vi "cycleAllNLMethods_invP.vi"() -> ()   [LabVIEW 2014]
uses:
  ICRMKinematics.llb/nloptIKParams.ctl
  02_optimalHome/homeBus.ctl
  ICRMKinematics.llb/jntLims.ctl
  CWrapATC3DG/Release/CWrapATC3DG.llb/ascSetup.ctl
  <vilib>/Analysis/Matrix/Datatypes/RealMatrix.ctl
  ICRMKinematics.llb/knPms11A.ctl
  <vilib>/Analysis/Matrix/NI_Matrix.lvlib
panel:
  out "results":T3(array[cluster])=[{"invParams"={"nlParams"={"maxIts"=100000.0, "maxTimeSec"=60.0, "nlMethod"=enum."GN_DIRECT", "errTol"=1e-09, "tolFun"=1e-09, "tolX"=1e-09}, "qp0"=[0.0, 0.0, 0.0, 1.0, 100.0], "q0dn"=[-0.4, -0.2, -0.2, -0.2, -10.0], "q0up"=[0.4, 0.2, 0.2, 0.2, 10.0], "kn0"={"tx01"=806.0, "ty01"=-66.0, "tz01"=-28.0, "ry01"=0.0, "rz01"=-0.24, "tx23"=8.2, "ry34"=0.0, "rz34"=0.0, "cathL"=98.0, "ry45"=0.0, "rz45"=0.0}, "knPM"={"tx01"=20.0, "ty01"=20.0, "tz01"=20.0, "ry01"=0.2, "rz01"=0.2, "tx23"=1.0, "ry34"=0.2, "rz34"=0.2, "cathL"=10.0, "ry45"=0.2, "rz45"=0.2}}, "qps0out"=[-0.014814814700095935, -0.0666666667240261, 0.06666666660930724, -0.19999999994264056, -3.3333333304653614], "kn"={"tx01"=820.7873799668292, "ty01"=-46.00000000573594, "tz01"=-8.000000005735945, "ry01"=-0.022222222164862783, "rz01"=-0.2029629629056035, "tx23"=9.199999999713203, "ry34"=0.19999999994264056, "rz34"=-0.19999999994264056, "cathL"=88.00000000286798, "ry45"=-0.007407407350047968, "rz45"=-0.06666666683874499}, "fmin"=78538.53053676435, "retCodeOut"=3}, {"invParams"={"nlParams"={"maxIts"=100000.0, "maxTimeSec"=60.0, "nlMethod"=enum."GN_DIRECT_L", "errTol"=1e-09, "tolFun"=1e-09, "tolX"=1e-09}, "qp0"=[0.0, 0.0, 0.0, 1.0, 100.0], "q0dn"=[-0.4, -0.2, -0.2, -0.2, -10.0], "q0up"=[0.4, 0.2, 0.2, 0.2, 10.0], "kn0"={"tx01"=806.0, "ty01"=-66.0, "tz01"=-28.0, "ry01"=0.0, "rz01"=-0.24, "tx23"=8.2, "ry34"=0.0, "rz34"=0.0, "cathL"=98.0, "ry45"=0.0, "rz45"=0.0}, "knPM"={"tx01"=20.0, "ty01"=20.0, "tz01"=20.0, "ry01"=0.2, "rz01"=0.2, "tx23"=1.0, "ry34"=0.2, "rz34"=0.2, "cathL"=10.0, "ry45"=0.2, "rz45"=0.2}}, "qps0out"=[-0.014814814700095935, -0.0666666667240261, 0.06666666660930724, -0.19999999994264056, -3.3333333304653614], "kn"={"tx01"=820.7873799668292, "ty01"=-46.00000000573594, "tz01"=-8.000000005735945, "ry01"=-0.022222222164862783, "rz01"=-0.2029629629056035, "tx23"=9.199999999713203, "ry34"=0.19999999994264056, "rz34"=-0.19999999994264056, "cathL"=88.00000000286798, "ry45"=-0.007407407350047968, "rz45"=-0.06666666683874499}, "fmin"=78538.53053676435, "retCodeOut"=3}, {"invParams"={"nlParams"={"maxIts"=100000.0, "maxTimeSec"=60.0, "nlMethod"=enum."GN_DIRECT_L_NOSCAL", "errTol"=1e-09, "tolFun"=1e-09, "tolX"=1e-09}, "qp0"=[0.0, 0.0, 0.0, 1.0, 100.0], "q0dn"=[-0.4, -0.2, -0.2, -0.2, -10.0], "q0up"=[0.4, 0.2, 0.2, 0.2, 10.0], "kn0"={"tx01"=806.0, "ty01"=-66.0, "tz01"=-28.0, "ry01"=0.0, "rz01"=-0.24, "tx23"=8.2, "ry34"=0.0, "rz34"=0.0, "cathL"=98.0, "ry45"=0.0, "rz45"=0.0}, "knPM"={"tx01"=20.0, "ty01"=20.0, "tz01"=20.0, "ry01"=0.2, "rz01"=0.2, "tx23"=1.0, "ry34"=0.2, "rz34"=0.2, "cathL"=10.0, "ry45"=0.2, "rz45"=0.2}}, "qps0out"=[-0.09053497938562868, 0.0222222222031024, 0.06666666664754684, -0.19999999998088017, -9.999999999964587], "kn"={"tx01"=825.835390946526, "ty01"=-61.30864197533225, "tz01"=-8.000000000023604, "ry01"=-0.03155006856798581, "rz01"=-0.20790123454878143, "tx23"=8.97777777780964, "ry34"=0.19999999998088017, "rz34"=-0.19999999998088017, "cathL"=107.7530864197885, "ry45"=-0.06666666664754684, "rz45"=-0.11111111116847056}, "fmin"=89200.3304411556, "retCodeOut"=3}, {"invParams"={"nlParams"={"maxIts"=100000.0, "maxTimeSec"=60.0, "nlMethod"=enum."GN_DIRECT_L_RAND", "errTol"=1e-09, "tolFun"=1e-09, "tolX"=1e-09}, "qp0"=[0.0, 0.0, 0.0, 1.0, 100.0], "q0dn"=[-0.4, -0.2, -0.2, -0.2, -10.0], "q0up"=[0.4, 0.2, 0.2, 0.2, 10.0], "kn0"={"tx01"=806.0, "ty01"=-66.0, "tz01"=-28.0, "ry01"=0.0, "rz01"=-0.24, "tx23"=8.2, "ry34"=0.0, "rz34"=0.0, "cathL"=98.0, "ry45"=0.0, "rz45"=0.0}, "knPM"={"tx01"=20.0, "ty01"=20.0, "tz01"=20.0, "ry01"=0.2, "rz01"=0.2, "tx23"=1.0, "ry34"=0.2, "rz34"=0.2, "cathL"=10.0, "ry45"=0.2, "rz45"=0.2}}, "qps0out"=[-0.044444441347034715, 0.03703703548833217, 0.1407407391920358, -0.1555555540068507, -9.999999922564756], "kn"={"tx01"=820.7325102364423, "ty01"=-46.00000015487049, "tz01"=-8.000000154870495, "ry01"=0.08148148303018635, "rz01"=-0.33629629784500115, "tx23"=8.75555554781203, "ry34"=0.06666666511796175, "rz34"=-0.11111111059487616, "cathL"=99.11111118854636, "ry45"=0.027160493310925515, "rz45"=-0.11111110956240623}, "fmin"=83347.32667099027, "retCodeOut"=3}, {"invParams"={"nlParams"={"maxIts"=100000.0, "maxTimeSec"=60.0, "nlMethod"=enum."GN_DIRECT_L_RAND_NOSCAL", "errTol"=1e-09, "tolFun"=1e-09, "tolX"=1e-09}, "qp0"=[0.0, 0.0, 0.0, 1.0, 100.0], "q0dn"=[-0.4, -0.2, -0.2, -0.2, -10.0], "q0up"=[0.4, 0.2, 0.2, 0.2, 10.0], "kn0"={"tx01"=806.0, "ty01"=-66.0, "tz01"=-28.0, "ry01"=0.0, "rz01"=-0.24, "tx23"=8.2, "ry34"=0.0, "rz34"=0.0, "cathL"=98.0, "ry45"=0.0, "rz45"=0.0}, "knPM"={"tx01"=20.0, "ty01"=20.0, "tz01"=20.0, "ry01"=0.2, "rz01"=0.2, "tx23"=1.0, "ry34"=0.2, "rz34"=0.2, "cathL"=10.0, "ry45"=0.2, "rz45"=0.2}}, "qps0out"=[-0.09053497938562868, 0.0222222222031024, 0.06666666664754684, -0.19999999998088017, -9.999999999964587], "kn"={"tx01"=825.835390946526, "ty01"=-61.30864197533225, "tz01"=-8.000000000023604, "ry01"=-0.03155006856798581, "rz01"=-0.20790123454878143, "tx23"=8.97777777780964, "ry34"=0.19999999998088017, "rz34"=-0.19999999998088017, "cathL"=107.7530864197885, "ry45"=-0.06666666664754684, "rz45"=-0.11111111116847056}, "fmin"=89200.3304411556, "retCodeOut"=3}, {"invParams"={"nlParams"={"maxIts"=100000.0, "maxTimeSec"=60.0, "nlMethod"=enum."GN_DIRECT_NOSCAL", "errTol"=1e-09, "tolFun"=1e-09, "tolX"=1e-09}, "qp0"=[0.0, 0.0, 0.0, 1.0, 100.0], "q0dn"=[-0.4, -0.2, -0.2, -0.2, -10.0], "q0up"=[0.4, 0.2, 0.2, 0.2, 10.0], "kn0"={"tx01"=806.0, "ty01"=-66.0, "tz01"=-28.0, "ry01"=0.0, "rz01"=-0.24, "tx23"=8.2, "ry34"=0.0, "rz34"=0.0, "cathL"=98.0, "ry45"=0.0, "rz45"=0.0}, "knPM"={"tx01"=20.0, "ty01"=20.0, "tz01"=20.0, "ry01"=0.2, "rz01"=0.2, "tx23"=1.0, "ry34"=0.2, "rz34"=0.2, "cathL"=10.0, "ry45"=0.2, "rz45"=0.2}}, "qps0out"=[-0.09053497938562868, 0.0222222222031024, 0.06666666664754684, -0.19999999998088017, -9.999999999964587], "kn"={"tx01"=825.835390946526, "ty01"=-61.30864197533225, "tz01"=-8.000000000023604, "ry01"=-0.03155006856798581, "rz01"=-0.20790123454878143, "tx23"=8.97777777780964, "ry34"=0.19999999998088017, "rz34"=-0.19999999998088017, "cathL"=107.7530864197885, "ry45"=-0.06666666664754684, "rz45"=-0.11111111116847056}, "fmin"=89200.3304411556, "retCodeOut"=3}, {"invParams"={"nlParams"={"maxIts"=100000.0, "maxTimeSec"=60.0, "nlMethod"=enum."GN_ESCH", "errTol"=1e-09, "tolFun"=1e-09, "tolX"=1e-09}, "qp0"=[0.0, 0.0, 0.0, 1.0, 100.0], "q0dn"=[-0.4, -0.2, -0.2, -0.2, -10.0], "q0up"=[0.4, 0.2, 0.2, 0.2, 10.0], "kn0"={"tx01"=806.0, "ty01"=-66.0, "tz01"=-28.0, "ry01"=0.0, "rz01"=-0.24, "tx23"=8.2, "ry34"=0.0, "rz34"=0.0, "cathL"=98.0, "ry45"=0.0, "rz45"=0.0}, "knPM"={"tx01"=20.0, "ty01"=20.0, "tz01"=20.0, "ry01"=0.2, "rz01"=0.2, "tx23"=1.0, "ry34"=0.2, "rz34"=0.2, "cathL"=10.0, "ry45"=0.2, "rz45"=0.2}}, "qps0out"=[-0.1496049559972273, 0.009381305080078096, 0.19794625178268757, -0.1998000520504, -9.963435211956861], "kn"={"tx01"=822.4184778784057, "ty01"=-47.011372142206795, "tz01"=-8.415394219210732, "ry01"=-0.04361262573634642, "rz01"=-0.272133169101733, "tx23"=9.183110023713372, "ry34"=0.19361551229581672, "rz34"=-0.19995700634438893, "cathL"=91.84527309696439, "ry45"=-0.011205503277072353, "rz45"=-0.06178247910138707}, "fmin"=71861.629220841, "retCodeOut"=6}, {"invParams"={"nlParams"={"maxIts"=100000.0, "maxTimeSec"=60.0, "nlMethod"=enum."GN_DIRECT", "errTol"=1e-09, "tolFun"=1e-09, "tolX"=1e-09}, "qp0"=[0.0, 0.0, 0.0, 1.0, 100.0], "q0dn"=[-0.4, -0.2, -0.2, -0.2, -10.0], "q0up"=[0.4, 0.2, 0.2, 0.2, 10.0], "kn0"={"tx01"=806.0, "ty01"=-66.0, "tz01"=-28.0, "ry01"=0.0, "rz01"=-0.24, "tx23"=8.2, "ry34"=0.0, "rz34"=0.0, "cathL"=98.0, "ry45"=0.0, "rz45"=0.0}, "knPM"={"tx01"=20.0, "ty01"=20.0, "tz01"=20.0, "ry01"=0.2, "rz01"=0.2, "tx23"=1.0, "ry34"=0.2, "rz34"=0.2, "cathL"=10.0, "ry45"=0.2, "rz45"=0.2}}, "qps0out"=[-0.014814814700095935, -0.0666666667240261, 0.06666666660930724, -0.19999999994264056, -3.3333333304653614], "kn"={"tx01"=820.7873799668292, "ty01"=-46.00000000573594, "tz01"=-8.000000005735945, "ry01"=-0.022222222164862783, "rz01"=-0.2029629629056035, "tx23"=9.199999999713203, "ry34"=0.19999999994264056, "rz34"=-0.19999999994264056, "cathL"=88.00000000286798, "ry45"=-0.007407407350047968, "rz45"=-0.06666666683874499}, "fmin"=78538.53053676435, "retCodeOut"=3}, {"invParams"={"nlParams"={"maxIts"=100000.0, "maxTimeSec"=60.0, "nlMethod"=enum."GN_ISRES", "errTol"=1e-09, "tolFun"=1e-09, "tolX"=1e-09}, "qp0"=[0.0, 0.0, 0.0, 1.0, 100.0], "q0dn"=[-0.4, -0.2, -0.2, -0.2, -10.0], "q0up"=[0.4, 0.2, 0.2, 0.2, 10.0], "kn0"={"tx01"=806.0, "ty01"=-66.0, "tz01"=-28.0, "ry01"=0.0, "rz01"=-0.24, "tx23"=8.2, "ry34"=0.0, "rz34"=0.0, "cathL"=98.0, "ry45"=0.0, "rz45"=0.0}, "knPM"={"tx01"=20.0, "ty01"=20.0, "tz01"=20.0, "ry01"=0.2, "rz01"=0.2, "tx23"=1.0, "ry34"=0.2, "rz34"=0.2, "cathL"=10.0, "ry45"=0.2, "rz45"=0.2}}, "qps0out"=[-0.15233500302423372, 0.001411312173998618, 0.1790954582443515, -0.19048957327232174, -9.500221765601044], "kn"={"tx01"=817.8395889157491, "ty01"=-49.80469334311147, "tz01"=-8.08345757827166, "ry01"=-0.02411683054361217, "rz01"=-0.2704187647515861, "tx23"=8.220218867165206, "ry34"=0.19769376826143897, "rz34"=-0.16858825923284948, "cathL"=98.42818791944134, "ry45"=-0.04229697037075319, "rz45"=0.0011992289937234136}, "fmin"=75766.64196993486, "retCodeOut"=6}, {"invParams"={"nlParams"={"maxIts"=100000.0, "maxTimeSec"=60.0, "nlMethod"=enum."GN_MLSL", "errTol"=1e-09, "tolFun"=1e-09, "tolX"=1e-09}, "qp0"=[0.0, 0.0, 0.0, 1.0, 100.0], "q0dn"=[-0.4, -0.2, -0.2, -0.2, -10.0], "q0up"=[0.4, 0.2, 0.2, 0.2, 10.0], "kn0"={"tx01"=806.0, "ty01"=-66.0, "tz01"=-28.0, "ry01"=0.0, "rz01"=-0.24, "tx23"=8.2, "ry34"=0.0, "rz34"=0.0, "cathL"=98.0, "ry45"=0.0, "rz45"=0.0}, "knPM"={"tx01"=20.0, "ty01"=20.0, "tz01"=20.0, "ry01"=0.2, "rz01"=0.2, "tx23"=1.0, "ry34"=0.2, "rz34"=0.2, "cathL"=10.0, "ry45"=0.2, "rz45"=0.2}}, "qps0out"=[-0.138430217866313, 0.051148661479379236, 0.2, -0.19999999999999993, -9.999999999999998], "kn"={"tx01"=823.8564738676603, "ty01"=-46.00000000000001, "tz01"=-8.0, "ry01"=-0.02592738205550581, "rz01"=-0.3127751385564531, "tx23"=9.2, "ry34"=0.2, "rz34"=-0.19999999999999998, "cathL"=91.1141365134803, "ry45"=-0.010452229236497568, "rz45"=-0.06809760694315031}, "fmin"=70534.84812392344, "retCodeOut"=6}, {"invParams"={"nlParams"={"maxIts"=100000.0, "maxTimeSec"=60.0, "nlMethod"=enum."GN_MLSL_LDS", "errTol"=1e-09, "tolFun"=1e-09, "tolX"=1e-09}, "qp0"=[0.0, 0.0, 0.0, 1.0, 100.0], "q0dn"=[-0.4, -0.2, -0.2, -0.2, -10.0], "q0up"=[0.4, 0.2, 0.2, 0.2, 10.0], "kn0"={"tx01"=806.0, "ty01"=-66.0, "tz01"=-28.0, "ry01"=0.0, "rz01"=-0.24, "tx23"=8.2, "ry34"=0.0, "rz34"=0.0, "cathL"=98.0, "ry45"=0.0, "rz45"=0.0}, "knPM"={"tx01"=20.0, "ty01"=20.0, "tz01"=20.0, "ry01"=0.2, "rz01"=0.2, "tx23"=1.0, "ry34"=0.2, "rz34"=0.2, "cathL"=10.0, "ry45"=0.2, "rz45"=0.2}}, "qps0out"=[-0.13829629157156895, 0.05150340426484309, 0.2, -0.2, -10.0], "kn"={"tx01"=823.8902581005755, "ty01"=-46.0, "tz01"=-8.0, "ry01"=-0.025883463083169713, "rz01"=-0.3129780965912823, "tx23"=9.2, "ry34"=0.2, "rz34"=-0.2, "cathL"=91.08907032219777, "ry45"=-0.010706972384393597, "rz45"=-0.1713198802142}, "fmin"=70547.2754347243, "retCodeOut"=6}, {"invParams"={"nlParams"={"maxIts"=100000.0, "maxTimeSec"=60.0, "nlMethod"=enum."GN_ORIG_DIRECT", "errTol"=1e-09, "tolFun"=1e-09, "tolX"=1e-09}, "qp0"=[0.0, 0.0, 0.0, 1.0, 100.0], "q0dn"=[-0.4, -0.2, -0.2, -0.2, -10.0], "q0up"=[0.4, 0.2, 0.2, 0.2, 10.0], "kn0"={"tx01"=806.0, "ty01"=-66.0, "tz01"=-28.0, "ry01"=0.0, "rz01"=-0.24, "tx23"=8.2, "ry34"=0.0, "rz34"=0.0, "cathL"=98.0, "ry45"=0.0, "rz45"=0.0}, "knPM"={"tx01"=20.0, "ty01"=20.0, "tz01"=20.0, "ry01"=0.2, "rz01"=0.2, "tx23"=1.0, "ry34"=0.2, "rz34"=0.2, "cathL"=10.0, "ry45"=0.2, "rz45"=0.2}}, "qps0out"=[-0.0237768632830361, -0.007376924249352235, 0.06663618350861152, -0.19996951684194483, -9.99847584209724], "kn"={"tx01"=821.558603871361, "ty01"=-46.003048315805515, "tz01"=-8.003048315805517, "ry01"=-0.02219173906416705, "rz01"=-0.24932784636488337, "tx23"=9.199847584209724, "ry34"=0.19996951684194483, "rz34"=-0.19996951684194483, "cathL"=94.66819082456944, "ry45"=-0.023959762231367157, "rz45"=-0.11114159426916628}, "fmin"=73491.99967495592, "retCodeOut"=6}, {"invParams"={"nlParams"={"maxIts"=100000.0, "maxTimeSec"=60.0, "nlMethod"=enum."GN_ORIG_DIRECT_L", "errTol"=1e-09, "tolFun"=1e-09, "tolX"=1e-09}, "qp0"=[0.0, 0.0, 0.0, 1.0, 100.0], "q0dn"=[-0.4, -0.2, -0.2, -0.2, -10.0], "q0up"=[0.4, 0.2, 0.2, 0.2, 10.0], "kn0"={"tx01"=806.0, "ty01"=-66.0, "tz01"=-28.0, "ry01"=0.0, "rz01"=-0.24, "tx23"=8.2, "ry34"=0.0, "rz34"=0.0, "cathL"=98.0, "ry45"=0.0, "rz45"=0.0}, "knPM"={"tx01"=20.0, "ty01"=20.0, "tz01"=20.0, "ry01"=0.2, "rz01"=0.2, "tx23"=1.0, "ry34"=0.2, "rz34"=0.2, "cathL"=10.0, "ry45"=0.2, "rz45"=0.2}}, "qps0out"=[-0.020739836769848852, -0.022222222222300903, 0.06666666666664055, -0.19999999999997378, -9.999999999998687], "kn"={"tx01"=820.7995732338909, "ty01"=-46.000000000002615, "tz01"=-8.000000000002615, "ry01"=-0.022222222222195987, "rz01"=-0.232592592592514, "tx23"=9.199999999999607, "ry34"=0.19999999999997387, "rz34"=-0.19999999999997378, "cathL"=94.66666666666798, "ry45"=-0.020454200603569617, "rz45"=-0.0666666666919237}, "fmin"=73530.37235081624, "retCodeOut"=6}, {"invParams"={"nlParams"={"maxIts"=100000.0, "maxTimeSec"=60.0, "nlMethod"=enum."LN_BOBYQA", "errTol"=1e-09, "tolFun"=1e-09, "tolX"=1e-09}, "qp0"=[0.0, 0.0, 0.0, 1.0, 100.0], "q0dn"=[-0.4, -0.2, -0.2, -0.2, -10.0], "q0up"=[0.4, 0.2, 0.2, 0.2, 10.0], "kn0"={"tx01"=806.0, "ty01"=-66.0, "tz01"=-28.0, "ry01"=0.0, "rz01"=-0.24, "tx23"=8.2, "ry34"=0.0, "rz34"=0.0, "cathL"=98.0, "ry45"=0.0, "rz45"=0.0}, "knPM"={"tx01"=20.0, "ty01"=20.0, "tz01"=20.0, "ry01"=0.2, "rz01"=0.2, "tx23"=1.0, "ry34"=0.2, "rz34"=0.2, "cathL"=10.0, "ry45"=0.2, "rz45"=0.2}}, "qps0out"=[-0.13843189384887258, 0.05114825382835384, 0.2, -0.2, -10.0], "kn"={"tx01"=823.8561446724875, "ty01"=-46.0, "tz01"=-8.0, "ry01"=-0.025927278051725504, "rz01"=-0.3127759414134171, "tx23"=9.2, "ry34"=0.2, "rz34"=-0.2, "cathL"=91.11430513275022, "ry45"=-0.010549435810457568, "rz45"=-0.06826506334333109}, "fmin"=70534.84805891909, "retCodeOut"=3}, {"invParams"={"nlParams"={"maxIts"=100000.0, "maxTimeSec"=60.0, "nlMethod"=enum."LN_COBYLA", "errTol"=1e-09, "tolFun"=1e-09, "tolX"=1e-09}, "qp0"=[0.0, 0.0, 0.0, 1.0, 100.0], "q0dn"=[-0.4, -0.2, -0.2, -0.2, -10.0], "q0up"=[0.4, 0.2, 0.2, 0.2, 10.0], "kn0"={"tx01"=806.0, "ty01"=-66.0, "tz01"=-28.0, "ry01"=0.0, "rz01"=-0.24, "tx23"=8.2, "ry34"=0.0, "rz34"=0.0, "cathL"=98.0, "ry45"=0.0, "rz45"=0.0}, "knPM"={"tx01"=20.0, "ty01"=20.0, "tz01"=20.0, "ry01"=0.2, "rz01"=0.2, "tx23"=1.0, "ry34"=0.2, "rz34"=0.2, "cathL"=10.0, "ry45"=0.2, "rz45"=0.2}}, "qps0out"=[-0.13843555082646675, 0.051142164081202264, 0.2, -0.2, -10.0], "kn"={"tx01"=823.8555250347629, "ty01"=-46.0, "tz01"=-8.0, "ry01"=-0.025926895334690593, "rz01"=-0.31277177020327096, "tx23"=9.2, "ry34"=0.2, "rz34"=-0.2, "cathL"=91.11476719455123, "ry45"=-0.011776126440051478, "rz45"=-0.06675896243504564}, "fmin"=70534.85238951069, "retCodeOut"=6}, {"invParams"={"nlParams"={"maxIts"=100000.0, "maxTimeSec"=60.0, "nlMethod"=enum."LN_NELDERMEAD", "errTol"=1e-09, "tolFun"=1e-09, "tolX"=1e-09}, "qp0"=[0.0, 0.0, 0.0, 1.0, 100.0], "q0dn"=[-0.4, -0.2, -0.2, -0.2, -10.0], "q0up"=[0.4, 0.2, 0.2, 0.2, 10.0], "kn0"={"tx01"=806.0, "ty01"=-66.0, "tz01"=-28.0, "ry01"=0.0, "rz01"=-0.24, "tx23"=8.2, "ry34"=0.0, "rz34"=0.0, "cathL"=98.0, "ry45"=0.0, "rz45"=0.0}, "knPM"={"tx01"=20.0, "ty01"=20.0, "tz01"=20.0, "ry01"=0.2, "rz01"=0.2, "tx23"=1.0, "ry34"=0.2, "rz34"=0.2, "cathL"=10.0, "ry45"=0.2, "rz45"=0.2}}, "qps0out"=[-0.13783975519613456, 0.05072994402657563, 0.19997508419385052, -0.19999914544377612, -9.999959686536547], "kn"={"tx01"=823.79240897062, "ty01"=-46.00044509553568, "tz01"=-8.000043635563326, "ry01"=-0.02541603371607614, "rz01"=-0.31245853621999065, "tx23"=9.198695981990365, "ry34"=0.2, "rz34"=-0.1999938142014731, "cathL"=91.15870639107467, "ry45"=0.0014237487464126306, "rz45"=-0.07574761531796181}, "fmin"=70536.64571685604, "retCodeOut"=6}, {"invParams"={"nlParams"={"maxIts"=100000.0, "maxTimeSec"=60.0, "nlMethod"=enum."LN_SBPLX", "errTol"=1e-09, "tolFun"=1e-09, "tolX"=1e-09}, "qp0"=[0.0, 0.0, 0.0, 1.0, 100.0], "q0dn"=[-0.4, -0.2, -0.2, -0.2, -10.0], "q0up"=[0.4, 0.2, 0.2, 0.2, 10.0], "kn0"={"tx01"=806.0, "ty01"=-66.0, "tz01"=-28.0, "ry01"=0.0, "rz01"=-0.24, "tx23"=8.2, "ry34"=0.0, "rz34"=0.0, "cathL"=98.0, "ry45"=0.0, "rz45"=0.0}, "knPM"={"tx01"=20.0, "ty01"=20.0, "tz01"=20.0, "ry01"=0.2, "rz01"=0.2, "tx23"=1.0, "ry34"=0.2, "rz34"=0.2, "cathL"=10.0, "ry45"=0.2, "rz45"=0.2}}, "qps0out"=[-0.13843066556684153, 0.05114778508914627, 0.2, -0.2, -10.0], "kn"={"tx01"=823.8563685030279, "ty01"=-46.0, "tz01"=-8.0, "ry01"=-0.025927516925628676, "rz01"=-0.3127743997607033, "tx23"=9.2, "ry34"=0.2, "rz34"=-0.2, "cathL"=91.11419845516922, "ry45"=-0.010609046883888796, "rz45"=-0.06828958285674085}, "fmin"=70534.84805164875, "retCodeOut"=4}]
  out "of":i32=17
  out "i":i32=16
  in  "data":T5(array[cluster])=[{"jointQps"=[0.0, 0.0, 0.0, 0.0, 100.0], "ascH05"=[[0.9907658398151398, -0.12067683041095734, 0.060893923044204774, 1012.972677731514], [-0.053780481219291736, 0.06135091185569776, 0.9966100752353668, -95.98322390317912], [-0.1240105926990509, -0.990737646818161, 0.054297372698784, -38.01717255115515], [0.0, 0.0, 0.0, 1.0]], "poseGRF"=[[-0.20091360807418823, -0.7534538060426712, 0.625877857208252, 795.8009765625], [-0.08737857639789592, -0.6225746273994446, -0.7775267362594604, -56.449121093749966], [0.9755924940109253, -0.21092700958251961, 0.059254452586173914, -53.29814453125005], [0.0, 0.0, 0.0, 1.0]]}, {"jointQps"=[0.0, 0.0, 0.0, 0.004016064257028112, 100.0], "ascH05"=[[0.9905737936496735, -0.1201397031545639, 0.06117585301399237, 1012.9534731149673], [-0.05397139489650731, 0.06231847405433667, 0.996301144361496, -96.11393636465073], [-0.12354400753974915, -0.9905025660991669, 0.05526317656040204, -38.19375622272497], [0.0, 0.0, 0.0, 1.0]], "poseGRF"=[[-0.20109128952026367, -0.7539264261722565, 0.6250251531600952, 795.68935546875], [-0.08786582946777355, -0.6216026544570923, -0.7780674397945404, -56.33749999999998], [0.9753671586513519, -0.21143388748168954, 0.05876922607421865, -53.40976562500005], [0.0, 0.0, 0.0, 1.0]]}, {"jointQps"=[0.0, 0.0, 0.0, 0.008032128514056224, 100.0], "ascH05"=[[0.9907330870628357, -0.1195027232170105, 0.061807125806808534, 1012.8577813625335], [-0.054564446210861255, 0.06295019388198866, 0.9963498711585999, -96.06162040233608], [-0.12297862768173218, -0.9906611144542694, 0.05585592985153211, -38.24883933067328], [0.0, 0.0, 0.0, 1.0]], "poseGRF"=[[-0.20146149396896362, -0.7531874477863312, 0.6259616017341614, 795.91259765625], [-0.0888538956642152, -0.6223757863044739, -0.7774698436260223, -56.33749999999998], [0.9753072559833527, -0.21228057146072396, 0.058469712734222315, -53.74462890625005], [0.0, 0.0, 0.0, 1.0]]}, {"jointQps"=[0.0, 0.0, 0.0, 0.012048192771084338, 100.0], "ascH05"=[[0.990741491317749, -0.11875051259994507, 0.06274437904357916, 1012.5237585067749], [-0.05557483434677129, 0.06274437904357924, 0.996284008026123, -96.16265921592708], [-0.12227010726928711, -0.990741491317749, 0.055574834346771365, -38.06636619567877], [0.0, 0.0, 0.0, 1.0]], "poseGRF"=[[-0.2015436589717865, -0.7535777539014816, 0.6253535449504852, 795.8009765625], [-0.08861736953258526, -0.621805876493454, -0.777862936258316, -56.449121093749966], [0.9752402007579803, -0.21223655343055733, 0.05855365097522726, -53.74462890625005], [0.0, 0.0, 0.0, 1.0]]}, {"jointQps"=[0.0, 0.0, 0.0, 0.01606425702811245, 100.0], "ascH05"=[[0.9908362030982971, -0.11802774667739868, 0.06179282069206244, 1012.6448507785797], [-0.05457875132560735, 0.06339436769485488, 0.9962467551231384, -95.9514298200607], [-0.121532142162323, -0.9907350242137909, 0.05638557672500623, -38.215811872482355], [0.0, 0.0, 0.0, 1.0]], "poseGRF"=[[-0.20161235332489014, -0.7529065757989883, 0.6261700391769409, 796.13583984375], [-0.0884058326482774, -0.6226986646652222, -0.7771972417831421, -56.560742187499955], [0.9752649068832397, -0.2120915651321412, 0.05899406969547262, -53.633007812500054], [0.0, 0.0, 0.0, 1.0]]}, {"jointQps"=[0.0, 0.0, 0.0, 0.020080321285140562, 100.0], "ascH05"=[[0.9907293021678925, -0.11835725605487823, 0.0617447197437287, 1012.8574028730392], [-0.05437628924846654, 0.06448951363563551, 0.9961173236370087, -96.0428047060966], [-0.12191829085350037, -0.9905544221401215, 0.05747406184673322, -38.58929002285009], [0.0, 0.0, 0.0, 1.0]], "poseGRF"=[[-0.20159786939620972, -0.7524719685316086, 0.6268618702888489, 796.35908203125], [-0.08795742690563213, -0.623507559299469, -0.7767325043678284, -56.560742187499955], [0.9754144549369812, -0.2117447257041932, 0.05951790511608114, -53.52138671875005], [0.0, 0.0, 0.0, 1.0]]}, {"jointQps"=[0.0, 0.0, 0.0, 0.024096385542168676, 100.0], "ascH05"=[[0.9907698333263397, -0.11849133670330048, 0.06288805603981024, 1012.526592707634], [-0.05518047511577611, 0.06723341345787062, 0.9960194528102875, -96.2348443865776], [-0.1222710907459259, -0.9904844462871552, 0.06008584797382367, -39.18267548084265], [0.0, 0.0, 0.0, 1.0]], "poseGRF"=[[-0.20138800144195557, -0.7531352341175079, 0.6260890960693359, 796.13583984375], [-0.08704555034637462, -0.6228947639465332, -0.7772918045520782, -56.449121093749966], [0.9755118191242218, -0.21106112003326424, 0.05989372730255117, -53.18652343750005], [0.0, 0.0, 0.0, 1.0]]}, {"jointQps"=[0.0, 0.0, 0.0, 0.028112449799196786, 100.0], "ascH05"=[[0.9907981157302856, -0.11803437769412994, 0.06235623359680182, 1012.5294209480286], [-0.05473853647708898, 0.06670272350311293, 0.9960199594497681, -95.96740833520886], [-0.12175428867340088, -0.9905149936676025, 0.059642776846885806, -38.907753086090146], [0.0, 0.0, 0.0, 1.0]], "poseGRF"=[[-0.2016635537147522, -0.7530561536550522, 0.6262139081954956, 796.13583984375], [-0.08679892122745525, -0.6230931878089905, -0.7772557139396667, -56.449121093749966], [0.9755528569221497, -0.21110880374908456, 0.06029357016086569, -53.18652343750005], [0.0, 0.0, 0.0, 1.0]]}, {"jointQps"=[0.0, 0.0, 0.0, 0.0321285140562249, 100.0], "ascH05"=[[0.9908184707164764, -0.1173403412103653, 0.062031239271164, 1012.6430775403976], [-0.054576650261879016, 0.06569287180900588, 0.9960139095783234, -95.72797752618789], [-0.12098768353462219, -0.9905824363231659, 0.05870510637760175, -38.719471478462275], [0.0, 0.0, 0.0, 1.0]], "poseGRF"=[[-0.20105329155921936, -0.7528541088104248, 0.6264556646347046, 796.35908203125], [-0.08644366264343273, -0.6233826577663422, -0.7769041061401367, -56.449121093749966], [0.9755836725234985, -0.21038818359375008, 0.06026396155357351, -53.18652343750005], [0.0, 0.0, 0.0, 1.0]]}, {"jointQps"=[0.0, 0.0, 0.0, 0.03614457831325301, 100.0], "ascH05"=[[0.991156131029129, -0.11538432538509369, 0.06270787119865423, 1012.5652224779129], [-0.05537511408329015, 0.06568643450737013, 0.9961200654506683, -95.91944500207899], [-0.11907735466957092, -0.9909631907939911, 0.0587267726659776, -38.30519640445715], [0.0, 0.0, 0.0, 1.0]], "poseGRF"=[[-0.2015078067779541, -0.752620205283165, 0.6264599561691284, 796.2474609375], [-0.08715771138668071, -0.6232631206512451, -0.7768148183822632, -56.33749999999998], [0.9753423929214478, -0.21118843555450448, 0.060010895133018397, -53.29814453125005], [0.0, 0.0, 0.0, 1.0]]}, {"jointQps"=[0.0, 0.0, 0.0, 0.040160642570281124, 100.0], "ascH05"=[[0.9909386932849884, -0.11602163314819336, 0.0629947185516358, 1012.4318576097488], [-0.055811405181884814, 0.06413987278938307, 0.9960722923278809, -95.96307411193845], [-0.11964297294616699, -0.9908652305603027, 0.05710080265998853, -38.13851604461676], [0.0, 0.0, 0.0, 1.0]], "poseGRF"=[[-0.20116353034973145, -0.7533643990755081, 0.6260089874267578, 796.13583984375], [-0.08568505942821514, -0.6230900287628174, -0.7773858904838562, -56.33749999999998], [0.9757577776908875, -0.21003055572509774, 0.06079359352588644, -52.96328125000005], [0.0, 0.0, 0.0, 1.0]]}, {"jointQps"=[0.0, 0.0, 0.0, 0.04417670682730924, 100.0], "ascH05"=[[0.9911193251609802, -0.1161518543958664, 0.0619714260101319, 1012.673162984848], [-0.054650738835334826, 0.06517785787582411, 0.9961999654769897, -95.84700747728346], [-0.11977064609527588, -0.9909136295318604, 0.058261469006538516, -38.374525547027645], [0.0, 0.0, 0.0, 1.0]], "poseGRF"=[[-0.2014598846435547, -0.7540600448846817, 0.6249626278877258, 795.91259765625], [-0.08384202420711528, -0.6224267482757568, -0.7780272364616394, -56.22587890624999], [0.9757844805717468, -0.20916336774826058, 0.062179222702979944, -52.62841796875005], [0.0, 0.0, 0.0, 1.0]]}, {"jointQps"=[0.0, 0.0, 0.0, 0.04819277108433735, 100.0], "ascH05"=[[0.9911406338214874, -0.11541353166103363, 0.062421351671218935, 1012.4520516633987], [-0.0551746934652329, 0.06494167447090163, 0.9961499869823456, -95.78778184652327], [-0.11904814839363098, -0.9909786880016327, 0.05801071226596845, -38.302275776863155], [0.0, 0.0, 0.0, 1.0]], "poseGRF"=[[-0.2010846734046936, -0.7546849399805069, 0.6243513822555542, 795.91259765625], [-0.0828918367624284, -0.6219744086265564, -0.778508722782135, -56.22587890624999], [0.975957453250885, -0.20832073688507088, 0.06251858174800863, -52.516796875000054], [0.0, 0.0, 0.0, 1.0]]}, {"jointQps"=[0.0, 0.0, 0.0, 0.05220883534136546, 100.0], "ascH05"=[[0.9913042187690735, -0.11406615376472473, 0.06321448087692266, 1012.2451679706573], [-0.056093156337738086, 0.06459027528762831, 0.9961791336536407, -95.99124922752378], [-0.11773154139518738, -0.9912155270576477, 0.057639181613922244, -37.947372889518796], [0.0, 0.0, 0.0, 1.0]], "poseGRF"=[[-0.20128950476646423, -0.7547886967658997, 0.6239610314369202, 795.8009765625], [-0.08076041936874401, -0.6220413744449615, -0.7785198092460632, -56.33749999999998], [0.97596675157547, -0.2071457505226136, 0.06426778435707083, -52.07031250000005], [0.0, 0.0, 0.0, 1.0]]}, {"jointQps"=[0.0, 0.0, 0.0, 0.05622489959839357, 100.0], "ascH05"=[[0.9915380775928497, -0.11230574548244476, 0.06201741099357611, 1012.268553853035], [-0.05510602891445165, 0.06362417340278638, 0.9962538778781891, -95.55767320394511], [-0.11585363745689392, -0.9914362728595734, 0.05690826475620282, -37.42471921443945], [0.0, 0.0, 0.0, 1.0]], "poseGRF"=[[-0.20185309648513794, -0.7550652921199799, 0.6235167384147644, 795.68935546875], [-0.08071511983871471, -0.6216302514076233, -0.7789109647274017, -56.33749999999998], [0.9759005010128021, -0.20759004354476937, 0.06454437971115103, -52.18193359375005], [0.0, 0.0, 0.0, 1.0]]}, {"jointQps"=[0.0, 0.0, 0.0, 0.060240963855421686, 100.0], "ascH05"=[[0.9915724694728851, -0.11158241331577301, 0.061981409788131776, 1012.2719930410385], [-0.055142030119895984, 0.063359171152115, 0.9962194859981537, -95.6728944182396], [-0.11511597037315369, -0.9914853870868683, 0.05668626725673688, -37.46257359981543], [0.0, 0.0, 0.0, 1.0]], "poseGRF"=[[-0.201692134141922, -0.7551415115594864, 0.6233542859554291, 795.68935546875], [-0.08063890039920818, -0.6214692890644073, -0.7789494693279266, -56.33749999999998], [0.9758619964122772, -0.20742759108543404, 0.0644681602716445, -52.18193359375005], [0.0, 0.0, 0.0, 1.0]]}, {"jointQps"=[0.0, 0.0, 0.0, 0.0642570281124498, 100.0], "ascH05"=[[0.9917207360267639, -0.11075133085250854, 0.062046617269516054, 1012.1751986026763], [-0.055327504873275805, 0.06273585557937635, 0.9963075518608093, -95.69144189357758], [-0.11425632238388062, -0.9916773736476898, 0.0560993552207948, -37.15336661338812], [0.0, 0.0, 0.0, 1.0]], "poseGRF"=[[-0.2022688388824463, -0.754878044128418, 0.6239188313484192, 795.91259765625], [-0.08162927627563488, -0.621874988079071, -0.7788686752319336, -56.22587890624999], [0.9759365916252136, -0.2084679603576661, 0.06416487693786611, -52.40517578125005], [0.0, 0.0, 0.0, 1.0]]}, {"jointQps"=[0.0, 0.0, 0.0, 0.06827309236947791, 100.0], "ascH05"=[[0.9918117523193359, -0.11005741357803345, 0.06057739257812506, 1012.2959213256836], [-0.053874552249908496, 0.06287574768066419, 0.9963016510009766, -95.32290444374081], [-0.11348915100097656, -0.991668701171875, 0.05644649267196668, -37.07664947509772], [0.0, 0.0, 0.0, 1.0]], "poseGRF"=[[-0.20267677307128906, -0.7546029090881348, 0.6240445077419281, 796.13583984375], [-0.08198133111000072, -0.6219578981399536, -0.7787055969238281, -56.22587890624999], [0.9757746458053589, -0.2089923322200776, 0.06419515609741201, -52.516796875000054], [0.0, 0.0, 0.0, 1.0]]}, {"jointQps"=[0.0, 0.0, 0.0, 0.07228915662650602, 100.0], "ascH05"=[[0.9921415746212006, -0.10817205905914307, 0.05997169017791754, 1012.1056613683701], [-0.05352008342742925, 0.06158241629600538, 0.9964867830276489, -95.51069974899292], [-0.11150515079498291, -0.9920428991317749, 0.055318981409073, -36.655007266998346], [0.0, 0.0, 0.0, 1.0]], "poseGRF"=[[-0.20288702845573425, -0.754681408405304, 0.6237607598304749, 796.0242187499999], [-0.08238154649734508, -0.6215948760509491, -0.7788566946983337, -56.33749999999998], [0.9756202101707458, -0.20942884683609017, 0.06394860148429861, -52.516796875000054], [0.0, 0.0, 0.0, 1.0]]}, {"jointQps"=[0.0, 0.0, 0.0, 0.07630522088353414, 100.0], "ascH05"=[[0.9928025305271149, -0.10459105670452118, 0.05504986643791205, 1012.3949991464615], [-0.04896275699138646, 0.05989268422126783, 0.9968160092830658, -94.3852405428886], [-0.10757520794868469, -0.9925221502780914, 0.054350689053535586, -36.038770794868526], [0.0, 0.0, 0.0, 1.0]], "poseGRF"=[[-0.20316895842552185, -0.7540903687477112, 0.6242943406105042, 796.13583984375], [-0.08257073163986217, -0.6221250593662262, -0.7783417105674744, -56.449121093749966], [0.9754884839057922, -0.20971757173538216, 0.0641411840915679, -52.62841796875005], [0.0, 0.0, 0.0, 1.0]]}, {"jointQps"=[0.0, 0.0, 0.0, 0.08032128514056225, 100.0], "ascH05"=[[0.9929757714271545, -0.10324347019195557, 0.055617213249206605, 1011.7425966739654], [-0.04961979389190679, 0.0597714185714723, 0.9968543648719788, -94.33932313919064], [-0.10625612735748291, -0.9927343726158142, 0.05423533916473401, -35.90686273574835], [0.0, 0.0, 0.0, 1.0]], "poseGRF"=[[-0.20309564471244812, -0.7546451091766357, 0.62380051612854, 796.0242187499999], [-0.08281970024108898, -0.6215551197528839, -0.778892993927002, -56.33749999999998], [0.9755804538726807, -0.20986700057983407, 0.06373998522758474, -52.74003906250005], [0.0, 0.0, 0.0, 1.0]]}, {"jointQps"=[0.0, 0.0, 0.0, 0.08433734939759036, 100.0], "ascH05"=[[0.9931384027004242, -0.10172475874423981, 0.05511501431465155, 1010.8658910512924], [-0.04939757287502294, 0.05788698792457594, 0.9969545900821686, -94.42872213125224], [-0.10462060570716858, -0.9929806888103485, 0.052472457289695865, -35.40844728946691], [0.0, 0.0, 0.0, 1.0]], "poseGRF"=[[-0.20290446281433105, -0.7544861286878586, 0.6238002181053162, 796.0242187499999], [-0.08330385386943828, -0.6214406490325928, -0.7787286043167114, -56.33749999999998], [0.9754160642623901, -0.21002012491226205, 0.06325583159923544, -52.85166015625005], [0.0, 0.0, 0.0, 1.0]]}, {"jointQps"=[0.0, 0.0, 0.0, 0.08835341365461848, 100.0], "ascH05"=[[0.9932567179203033, -0.10108165442943573, 0.05192771553993231, 1011.1009647607804], [-0.046250775456428576, 0.05770489573478712, 0.9969974458217621, -93.66755801439285], [-0.10380199551582336, -0.992937833070755, 0.05265454947948468, -35.214965176582396], [0.0, 0.0, 0.0, 1.0]], "poseGRF"=[[-0.20262515544891357, -0.7543348073959351, 0.6243223547935486, 796.13583984375], [-0.08362686634063732, -0.6218885779380798, -0.7785354852676392, -56.33749999999998], [0.9756054282188416, -0.20997607707977303, 0.06293213367462148, -52.85166015625005], [0.0, 0.0, 0.0, 1.0]]}, {"jointQps"=[0.0, 0.0, 0.0, 0.09236947791164658, 100.0], "ascH05"=[[0.993652880191803, -0.09868684411048889, 0.05053108930587775, 1011.1405809879303], [-0.04547244310379033, 0.052845537662506235, 0.9973856508731842, -93.254861497879], [-0.10111746191978455, -0.9935324788093567, 0.04803127050399793, -33.71867978572851], [0.0, 0.0, 0.0, 1.0]], "poseGRF"=[[-0.20217332243919373, -0.7547992318868637, 0.6236723363399506, 796.0242187499999], [-0.08283720910549175, -0.6213599145412445, -0.7788536250591278, -56.33749999999998], [0.9756162464618683, -0.20917239785194405, 0.06311072409152975, -52.74003906250005], [0.0, 0.0, 0.0, 1.0]]}, {"jointQps"=[0.0, 0.0, 0.0, 0.0963855421686747, 100.0], "ascH05"=[[0.9936568439006805, -0.09784950315952301, 0.04850217700004584, 1011.1409773588181], [-0.043353453278541614, 0.054058998823166025, 0.9972356855869293, -92.81972032785416], [-0.10023704171180725, -0.9933700263500214, 0.04949177801609052, -33.85387995243078], [0.0, 0.0, 0.0, 1.0]], "poseGRF"=[[-0.20249488949775696, -0.7546465247869492, 0.6239975392818451, 796.0242187499999], [-0.0829899162054063, -0.6216814815998077, -0.7787767946720123, -56.22587890624999], [0.9756930768489838, -0.20949760079383858, 0.0632634311914443, -52.74003906250005], [0.0, 0.0, 0.0, 1.0]]}, {"jointQps"=[0.0, 0.0, 0.0, 0.10040160642570281, 100.0], "ascH05"=[[0.9937727153301239, -0.09901487827301025, 0.04621255397796637, 1011.4874277830123], [-0.04101908206939702, 0.053849250078201426, 0.9974675178527832, -92.5862832069397], [-0.10127675533294678, -0.9933881759643555, 0.049464195966720706, -33.84623022079474], [0.0, 0.0, 0.0, 1.0]], "poseGRF"=[[-0.20249032974243164, -0.7552739381790161, 0.623264878988266, 795.91259765625], [-0.08251604437828075, -0.6210265159606934, -0.7793698310852051, -56.22587890624999], [0.9757504463195801, -0.2092546522617341, 0.06343281269073477, -52.74003906250005], [0.0, 0.0, 0.0, 1.0]]}, {"jointQps"=[0.0, 0.0, 0.0, 0.10441767068273092, 100.0], "ascH05"=[[0.9939553141593933, -0.09875182807445526, 0.043117046356201234, 1011.7289298534394], [-0.03802795708179479, 0.05283898115158094, 0.997657299041748, -92.28717070817947], [-0.10082101821899414, -0.9934859275817871, 0.048775032162666446, -33.800656509399474], [0.0, 0.0, 0.0, 1.0]], "poseGRF"=[[-0.20252695679664612, -0.7549966722726822, 0.6235119998455048, 796.0242187499999], [-0.08239139616489422, -0.6213115751743317, -0.7790943086147308, -56.33749999999998], [0.9757042825222015, -0.20918008685112008, 0.06363333761692037, -52.74003906250005], [0.0, 0.0, 0.0, 1.0]]}, {"jointQps"=[0.0, 0.0, 0.0, 0.10843373493975904, 100.0], "ascH05"=[[0.9942052364349365, -0.09838449954986572, 0.04142233729362494, 1011.7539220809937], [-0.036072224378585864, 0.05554592609405531, 0.9977238178253174, -92.09159743785858], [-0.10046947002410889, -0.9935162365436554, 0.05167925357818616, -34.211986064910946], [0.0, 0.0, 0.0, 1.0]], "poseGRF"=[[-0.20257484912872314, -0.7550368010997772, 0.6233891248703003, 795.91259765625], [-0.08275318145751964, -0.6211110353469849, -0.7791688740253448, -56.33749999999998], [0.9756262004375458, -0.20945560932159432, 0.06334829330444326, -52.74003906250005], [0.0, 0.0, 0.0, 1.0]]}, {"jointQps"=[0.0, 0.0, 0.0, 0.11244979919678715, 100.0], "ascH05"=[[0.9942961931228638, -0.09667390584945679, 0.041388392448425355, 1011.2049122810364], [-0.03610616922378545, 0.05575644969940199, 0.9976328611373901, -92.20661301612853], [-0.09876835346221924, -0.9935940504074097, 0.05195611715316785, -34.04187440872198], [0.0, 0.0, 0.0, 1.0]], "poseGRF"=[[-0.20232772827148438, -0.755235567688942, 0.6234257221221924, 795.91259765625], [-0.08247767388820659, -0.6211891174316406, -0.7792935371398926, -56.33749999999998], [0.9758267402648926, -0.2090938091278077, 0.06339444220066061, -52.74003906250005], [0.0, 0.0, 0.0, 1.0]]}, {"jointQps"=[0.0, 0.0, 0.0, 0.11646586345381527, 100.0], "ascH05"=[[0.9944072663784027, -0.09648972749710083, 0.038285315036773744, 1011.5508828878402], [-0.03287321329116826, 0.057058900594711436, 0.9976399540901184, -91.66007523536678], [-0.09846514463424683, -0.9935068488121033, 0.053577989339828616, -34.458037900924744], [0.0, 0.0, 0.0, 1.0]], "poseGRF"=[[-0.20222938060760498, -0.7544398307800293, 0.6241273880004883, 796.13583984375], [-0.08166551589965831, -0.6220835447311401, -0.7784304618835449, -56.22587890624999], [0.9757280349731445, -0.20843172073364266, 0.06420433521270742, -52.516796875000054], [0.0, 0.0, 0.0, 1.0]]}, {"jointQps"=[0.0, 0.0, 0.0, 0.12048192771084337, 100.0], "ascH05"=[[0.9945012927055359, -0.0969560295343399, 0.035892665386200014, 1011.6719066143036], [-0.03063975274562841, 0.05512732267379774, 0.997869610786438, -91.3251080870628], [-0.09874188899993896, -0.9936206936836243, 0.05186070501804364, -34.150849056243956], [0.0, 0.0, 0.0, 1.0]], "poseGRF"=[[-0.2026660442352295, -0.7542854845523834, 0.6244144439697266, 796.13583984375], [-0.08149492740631115, -0.6224431991577148, -0.7783550322055817, -56.33749999999998], [0.9758066236972809, -0.20864176750183114, 0.06468045711517324, -52.40517578125005], [0.0, 0.0, 0.0, 1.0]]}, {"jointQps"=[0.0, 0.0, 0.0, 0.12449799196787148, 100.0], "ascH05"=[[0.9946300983428955, -0.09579448401927948, 0.03322643041610724, 1011.9080293655395], [-0.027944400906562857, 0.05595183372497572, 0.9978266954421997, -90.83233071565627], [-0.0974663496017456, -0.9936107993125916, 0.05298586189746869, -34.35815839767462], [0.0, 0.0, 0.0, 1.0]], "poseGRF"=[[-0.2029498815536499, -0.7538092732429504, 0.6246243715286255, 796.2474609375], [-0.08164626359939586, -0.6226500272750854, -0.7779546976089478, -56.22587890624999], [0.9755603075027466, -0.20892870426177987, 0.06483489274978628, -52.40517578125005], [0.0, 0.0, 0.0, 1.0]]}, {"jointQps"=[0.0, 0.0, 0.0, 0.1285140562248996, 100.0], "ascH05"=[[0.9946471154689789, -0.09573227167129517, 0.02957969903945929, 1012.3562154531479], [-0.02403289079666143, 0.058566182851791514, 0.9976747632026672, -90.32955861091614], 
